vi "Stop Logging.vi"(8 "error in (no error)":errorcluster, 11 "Logger in.lvclass":refnum<class "Logger.lvclass">) -> (0 "error out":errorcluster, 3 "Logger out.lvclass":refnum<class "Logger.lvclass">)   [LabVIEW 2020, in "Logger.lvclass"]
uses:
  Logger.lvclass
  Logger.lvclass/Logger.ctl
  <vilib>/Skyline/TestMonitor/Shared/typedefs/Status Type.ctl
  <vilib>/Skyline/TestMonitor/Test Result/NI SystemLink Test Result.lvclass/NI SystemLink Test Result.ctl
  <vilib>/Skyline/TestMonitor/Test Result/Write Total Time In Seconds.vi
  <vilib>/Skyline/TestMonitor/Test Result/Update Test Result (Single).vi
  <vilib>/Skyline/TestMonitor/Shared/NI SystemLink Test Monitor.lvlib
  <vilib>/Skyline/TestMonitor/Test Result/NI SystemLink Test Result.lvclass
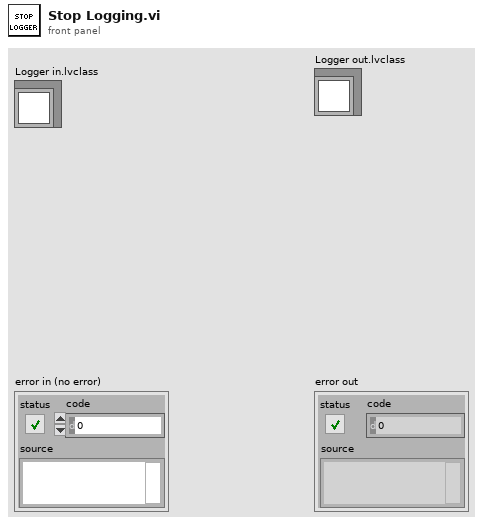
[diagram p1: front panel]
types:
  T1 = typedef "NI SystemLink Test Monitor.lvlib/Status Type.ctl" = enum16{"Failed", "Passed", "Looping", "Skipped", "Custom", "Done", "Running", "Waiting", "Terminated", "Errored", "Timed Out", "None"}
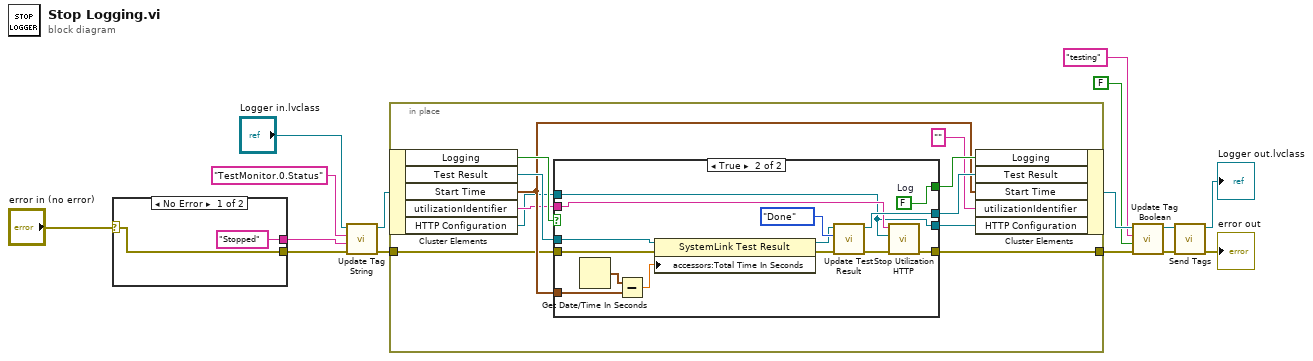
[diagram p0: block diagram]
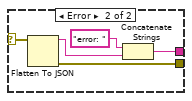
[diagram p2: hidden frame]
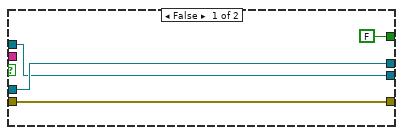
[diagram p3: hidden frame]
diagram:
  n1 = case shown="No Error" "error in (no error)" {
    selector: "error in (no error)" -> [w17 w22]
    tunnel: ["Stopped" ("JSON string") w18] -> w10
    tunnel: [w17 w21] -> w9
    frame No Error {
    }
    frame Error {
      n2 = Flatten To JSON(anything=w22) -> (JSON string=w19:string, 11:w21:errorcluster)  [unwired: 2 in]
      n3 = Concatenate Strings("error: " ("JSON string"), w19) -> (w18:string)
    }
  }
  n4 = call "Update Tag String.vi"("error in (no error)"=w9, "string"=w10, "Tag Path"="TestMonitor.0.Status", "Logger in.lvclass"="Logger in.lvclass") -> ("error out"=w5:errorcluster, "Logger out.lvclass"=w7:refnum<class "Logger.lvclass">)  [unwired: 6 in]
  n5 = in-place {
    in-place-border: [w33] -> w12
    in-place-border: w5 -> [w27]
    n6 = in-place-cluster #1(w7) -> ("Logging"=w29:bool, "Test Result"=w31:refnum<class "NI SystemLink Test Result.lvclass">, "Start Time"=w28:timestamp, "utilizationIdentifier"=w26:string, "HTTP Configuration"=w25:refnum<class "NI Skyline Configuration HTTP.lvclass">)
    n7 = case shown="True" w29 {
      tunnel: [w35 w39] -> w33
      tunnel: [w37 w51] -> w32
      tunnel: [FALSE ("Log") w50] -> w30
      tunnel: w31 -> [w37 w48]
      tunnel: w28 -> [_ w44]
      tunnel: w27 -> [w35 w42]
      tunnel: w26 -> [_ w41]
      tunnel: w25 -> [w34 w38]
      tunnel: [w34 w38] -> w23
      frame False {
      }
      frame True {
        w50 = FALSE  # Log
        n8 = Get Date/Time In Seconds() -> (seconds since 1Jan1904=w45:timestamp)
        n9 = Subtract(x=w45, y=w44) -> (x-y=w43:dbl)
        n10 = property on="Property Node" class="SystemLink Test Result"(reference=w48, error in=w42, "accessors:Total Time In Seconds"=w43) -> (reference out=w47:refnum<class "NI SystemLink Test Result.lvclass">, error out=w46:errorcluster)
        n11 = call-poly <vilib>:"Update Test Result.vi"("error in (no error)"=w46, "status type"=Status_Type."Done", "test result in"=w47) -> ("error out"=w40:errorcluster, "test result out"=w51:refnum<class "NI SystemLink Test Result.lvclass">)  [unwired: 7 in]
        n12 = call "Stop Utilization HTTP.vi"("error in (no error)"=w40, "configuration"=w38, "utilizationIdentifier"=w41) -> ("error out"=w39:errorcluster)  [unwired: 8 in]
      }
    }
    n13 = in-place-cluster #1("Logging"=w30, "Test Result"=w32, "Start Time"=w28, "utilizationIdentifier"="", "HTTP Configuration"=w23) -> (w15:refnum<class "Logger.lvclass">)
  }
  n14 = call "Update Tag Boolean.vi"("error in (no error)"=w12, "Value"=FALSE, "Tag Path"="testing", "Logger in.lvclass"=w15) -> ("error out"=w1:errorcluster, "Logger out.lvclass"=w2:refnum<class "Logger.lvclass">)  [unwired: 6 in]
  n15 = call "Send Tags.vi"("error in (no error)"=w1, "Logger in.lvclass"=w2) -> ("error out"=→"error out":errorcluster, "Logger out.lvclass"=→"Logger out.lvclass":refnum<class "Logger.lvclass">)  [unwired: 8 in]
